vi "Tutorial_6_ICP_IP_act_like_2_computer.vi"() -> ()   [LabVIEW 2020]
panel:
  in  "Text Server":string
  in  "?":bool
  out "Numeric 2":i32
  out "2 writte":i32
  out "error out":errorcluster
  out "String":string
  out "Numeric":i32
  out "Msg":string
  in  "Text":string
  out "1 write":i32
  out "error out 2":errorcluster
  in  "?":bool
  # "Client"
  # "Server"
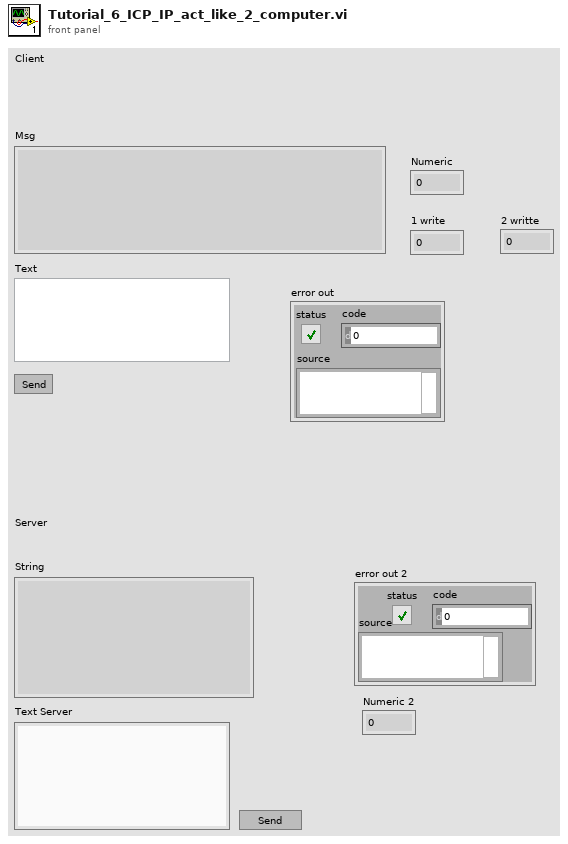
[diagram p1: front panel]
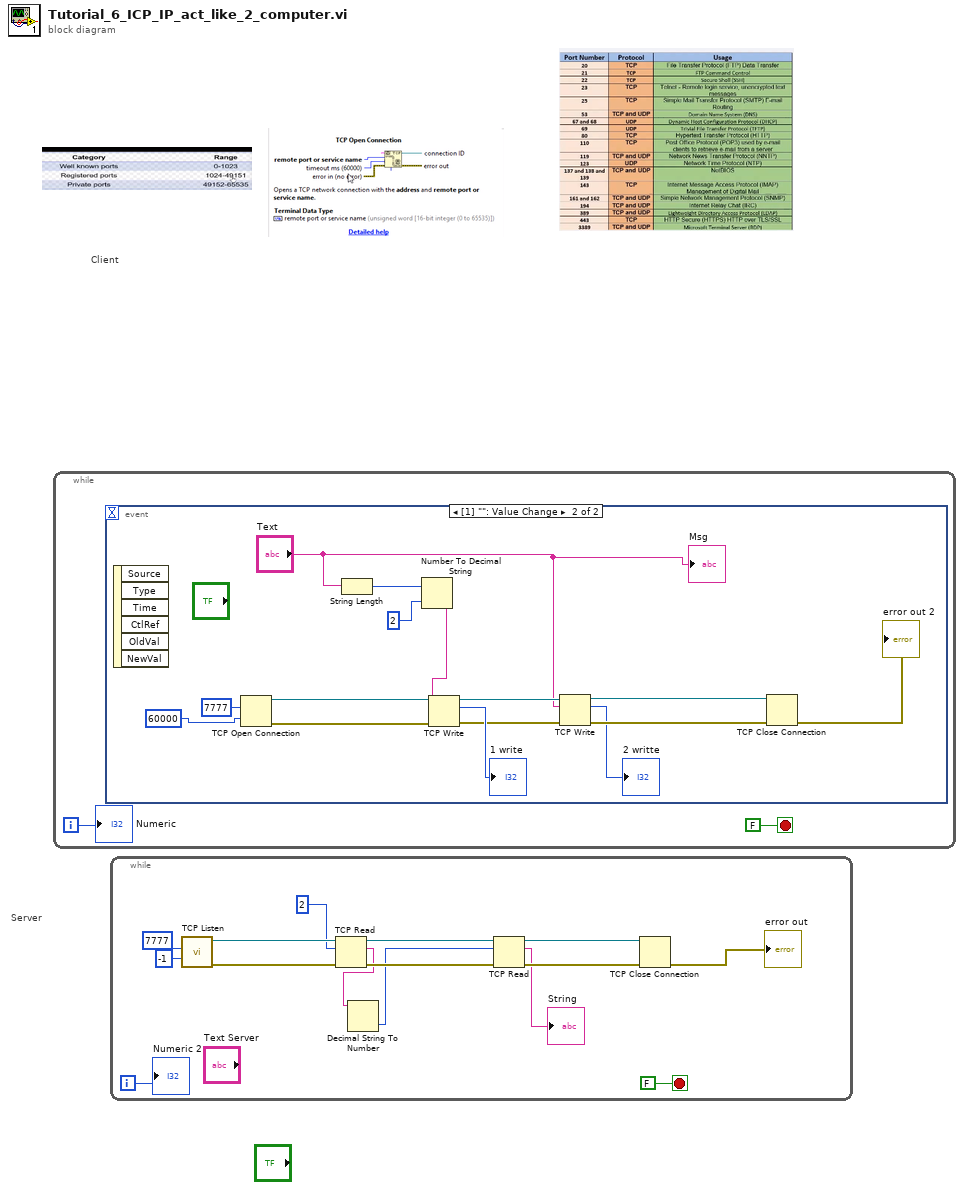
[diagram p0: block diagram]
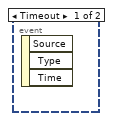
[diagram p2: hidden frame]
diagram:
  # "Server"
  # "Client"
  n1 = while {
    i -> [w1]
    stop <- FALSE stop-if-true
    n2 = event shown="[1] \"\": Value Change" {
      selector: _ -> [_ _]
      dyn-events: _ -> [_ _]
      timeout: _ -> [_ _]
      event Timeout {
        n3 = event-data() -> ()  [unwired: 1 in, 3 out]
      }
      event Value Change {
        n4 = event-data() -> ()  [unwired: 1 in, 6 out]
        n5 = TCP Open Connection(remote port or service name=u16 7777, timeout ms (60000)=60000) -> (connection ID=w14:refnum<k5>, error out=w15:errorcluster)  [unwired: 3 in]
        n6 = String Length(string="Text") -> (length=w6:i32)
        n7 = Number To Decimal String(number=w6, width (-)=i16 2) -> (decimal integer string=w5:string)
        n8 = TCP Write(connection ID=w14, data in=w5, error in (no error)=w15) -> (connection ID out=w11:refnum<k5>, bytes written=→"1 write":i32, error out=w8:errorcluster)  [unwired: 1 in]
        n9 = TCP Write(connection ID=w11, data in="Text", error in (no error)=w8) -> (connection ID out=w10:refnum<k5>, bytes written=→"2 writte":i32, error out=w9:errorcluster)  [unwired: 1 in]
        n10 = TCP Close Connection(connection ID=w10, error in (no error)=w9) -> (error out=→"error out 2":errorcluster)  [unwired: 1 in, 1 out]
        "Msg" <- "Text"
      }
    }
    "Numeric" <- w1
  }
  n11 = while {
    i -> [w18]
    stop <- FALSE stop-if-true
    n12 = call <vilib>:"TCP Listen.vi"("timeout ms (wait forever: -1)"=-1, "port"=u16 7777) -> ("error out"=w29:errorcluster, "connection ID"=w30:refnum<k5>)  [unwired: 5 in, 3 out]
    n13 = TCP Read(connection ID=w30, bytes to read=2, error in (no error)=w29) -> (connection ID out=w25:refnum<k5>, data out=w21:string, error out=w23:errorcluster)  [unwired: 2 in]
    n14 = Decimal String To Number(string=w21) -> (number=w20:i32)  [unwired: 2 in, 1 out]
    n15 = TCP Read(connection ID=w25, bytes to read=w20, error in (no error)=w23) -> (connection ID out=w24:refnum<k5>, data out=→"String":string, error out=w22:errorcluster)  [unwired: 2 in]
    n16 = TCP Close Connection(connection ID=w24, error in (no error)=w22) -> (error out=→"error out":errorcluster)  [unwired: 1 in, 1 out]
    "Numeric 2" <- w18
  }
